vi "Test SenseHat Lib.vi"() -> ()   [LabVIEW 2020]
uses:
  src/RPI.SenseHat/SenseHat/SenseHat.lvclass/SenseHat.ctl
  src/RPI.SenseHat/SenseHat/Get RPI.SenseHat.Display.vi
  <vilib>/MakerHub/LINX/Public/Utilities/Open Local.vi
  src/RPI.SenseHat.Display/Classes/SenseHat.Display/RPI.SenseHat.Display.lvclass
  src/RPI.SenseHat/SenseHat/SenseHat.lvclass
  <vilib>/MakerHub/LINX/LMH-LINX.lvlib
  src/RPI.SenseHat.Display/Classes/Color/Color.lvclass
  src/RPI.SenseHat.Display/RPI.SenseHat.Display.lvlib
panel:
  in  "Image":u32[][](array[colorbox])=[[0, 0, 0, 0, 0, 0, 0, 0], [0, 0, 0, 0, 0, 0, 0, 0], [0, 0, 0, 0, 0, 0, 0, 0], [0, 0, 0, 0, 0, 0, 0, 0], [0, 0, 0, 0, 0, 0, 0, 0], [0, 0, 0, 0, 0, 0, 0, 0], [0, 0, 0, 0, 0, 0, 0, 0], [0, 0, 0, 0, 0, 0, 0, 16777222]]
  in  "Color":u32(colorbox)
  in  "Actions":enum32{"reset", "clear", "fill", "draw"}(radio)
  out "Error Out":errorcluster
  out "Device Name":string
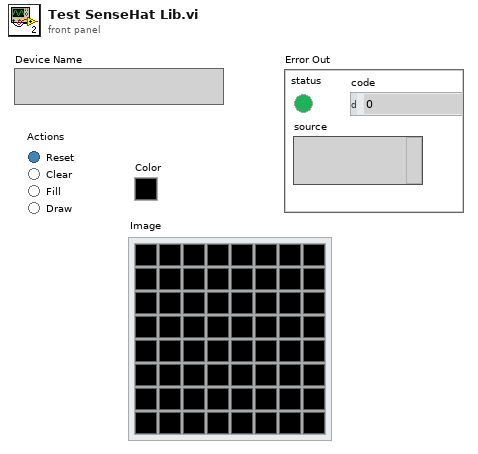
[diagram p1: front panel]
types:
  T1 = typedef "LMH-LINX.lvlib/LINX Ref.ctl" = cluster{"IO":T2, "Interface":T3, "LINX Device Config":T4}
  T2 = typedef "LMH-LINX.lvlib/Platform.ctl" = enum16{"Remote", "Local"}
  T3 = typedef "LMH-LINX.lvlib/Interface.ctl" = enum16{"Serial", "TCP"}
  T4 = typedef "LMH-LINX.lvlib/Device.lvlib/LINX Device Config.ctl" = cluster{"Interface":T3, "COM Port":refnum<visa-resource-name>, "TCP Configuration":T5, "Device Family":u8, "Device ID":u8, "Device Name":string, "TCP Ref":refnum<k5>, "Channels":T6}
  T5 = typedef "LMH-LINX.lvlib/Device.lvlib/TCP Config.ctl" = cluster{"IP Address":string, "Port":u16}
  T6 = typedef "LMH-LINX.lvlib/Channels.ctl" = cluster{"DI":u8[], "DO":u8[], "AI":u8[], "AO":u8[], "PWM":u8[], "QE":u8[], "UART":u8[], "I2C 2":u8[], "SPI":u8[], "CAN":u8[], "Servo":u8[], "AI Ref (V)":dbl, "AI Resolution (Bits)":u8, "AO Ref (V)":dbl, "AO Resolution (Bits)":u8}
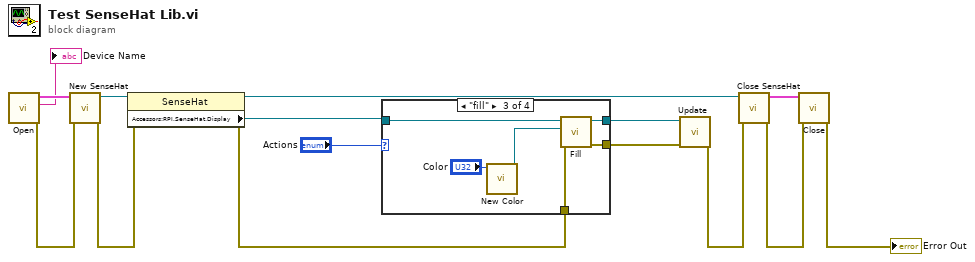
[diagram p0: block diagram]
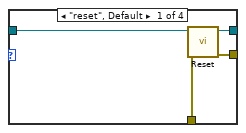
[diagram p2: hidden frame]
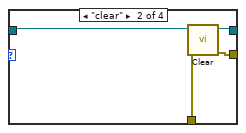
[diagram p3: hidden frame]
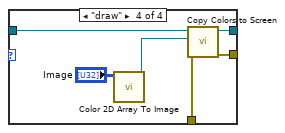
[diagram p4: hidden frame]
diagram:
  n1 = call-poly <vilib>:"Open.vi"() -> ("Error Out"=w5:errorcluster, "Device Name"=→"Device Name":string, "LINX Resource"=w15:T1)  [unwired: 9 in]
  n2 = call "New SenseHat.vi"("error in (no error)"=w5, "LINX Resource"=w15) -> ("error out"=w6:errorcluster, "SenseHat out"=w13:refnum<class "SenseHat.lvclass">)  [unwired: 8 in]
  n3 = property class="SenseHat"(reference=w13, error in=w6) -> (reference out=w12:refnum<class "SenseHat.lvclass">, error out=w4:errorcluster, "Accessors:RPI.SenseHat.Display"=w11:refnum<class "RPI.SenseHat.Display.lvclass">)
  n4 = case shown="\"fill\"" "Actions" {
    tunnel: w11 -> [w19 w23 w29 w34]
    tunnel: [w17 w22 w28 w33] -> w10
    tunnel: [w16 w21 w27 w32] -> w9
    tunnel: w4 -> [w18 w20 w26 w31]
    frame "reset", Default {
      n5 = call "Reset.vi"("error in (no error)"=w18, "senseHatDisplay in"=w19) -> ("error out"=w16:errorcluster, "senseHatDisplay out"=w17:refnum<class "RPI.SenseHat.Display.lvclass">)  [unwired: 8 in]
    }
    frame "clear" {
      n6 = call "Clear.vi"("error in (no error)"=w20, "senseHatDisplay in"=w23) -> ("error out"=w21:errorcluster, "senseHatDisplay out"=w22:refnum<class "RPI.SenseHat.Display.lvclass">)  [unwired: 8 in]
    }
    frame "fill" {
      n7 = call "New Color.vi"("Color Box"="Color") -> ("Color out"=w24:refnum<class "Color.lvclass">)  [unwired: 9 in, 1 out]
      n8 = call "Fill.vi"("error in (no error)"=w26, "Color"=w24, "senseHatDisplay in"=w29) -> ("error out"=w27:errorcluster, "senseHatDisplay out"=w28:refnum<class "RPI.SenseHat.Display.lvclass">)  [unwired: 7 in]
    }
    frame "draw" {
      n9 = call "Color 2D Array To Image.vi"("Color[]"="Image") -> ("Image out"=w30:refnum<class "Image.lvclass">)  [unwired: 9 in, 1 out]
      n10 = call "Copy Colors to Screen.vi"("error in (no error)"=w31, "Image"=w30, "senseHatDisplay in"=w34) -> ("error out"=w32:errorcluster, "senseHatDisplay out"=w33:refnum<class "RPI.SenseHat.Display.lvclass">)  [unwired: 7 in]
    }
  }
  n11 = call "Update.vi"("error in (no error)"=w9, "senseHatDisplay in"=w10) -> ("error out"=w8:errorcluster)  [unwired: 8 in, 1 out]
  n12 = call "Close SenseHat.vi"("error in (no error)"=w8, "SenseHat in"=w12) -> ("error out"=w7:errorcluster, "LINX Resource"=w14:T1)  [unwired: 8 in]
  n13 = call <vilib>:"Close.vi"("Error In"=w7, "LINX Resource"=w14) -> ("Error Out"=→"Error Out":errorcluster)  [unwired: 9 in]
